vi "ORGINAL_drawLabel.vi"(0 "reference":refnum<class "StateTransitionEdge.lvclass">, 1 "graphics":refnum<class "Graphics.lvclass">, 5 "error in (no error)":errorcluster) -> (14 "reference out":refnum<class "StateTransitionEdge.lvclass">, 19 "error out":errorcluster)   [LabVIEW 2012, in "StateTransitionEdge.lvclass"]
doc: "private void drawLabel(Graphics2D g2)"
uses:
  <resource>/Framework/Providers/Open_GDS/UML/StateTransitionEdge_class/StateTransitionEdge.lvclass
  <resource>/Framework/Providers/Open_GDS/UML/Graphics_class/Graphics.lvclass
  <resource>/Framework/Providers/Open_GDS/UML/General/Point/Point Point2D.ctl
  <resource>/Framework/Providers/Open_GDS/UML/SegmentedLineEdge_class/SegmentedLineEdge.lvclass
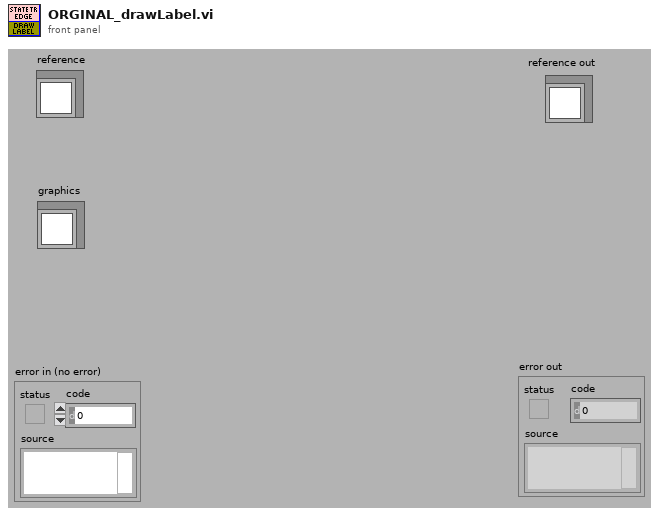
[diagram p1: front panel]
types:
  T1 = typedef "Point Point2D.ctl" = cluster{"x":dbl, "y":dbl}
  T2 = typedef "SegmentedLineEdge.lvclass/ObjectAttributes.ctl" = cluster{"lineStyle":refnum<class "LineStyle.lvclass">, "startArrowHead":refnum<class "ArrowHead.lvclass">, "endArrowHead":refnum<class "ArrowHead.lvclass">, "startLabel":string, "midLabel":string, "endLabel":string, "MidLabelOffset":T1, "SplitWire":bool}
  T3 = typedef "Rectangle Rectangle2D.ctl" = cluster{"x":dbl, "y":dbl, "width":dbl, "height":dbl}
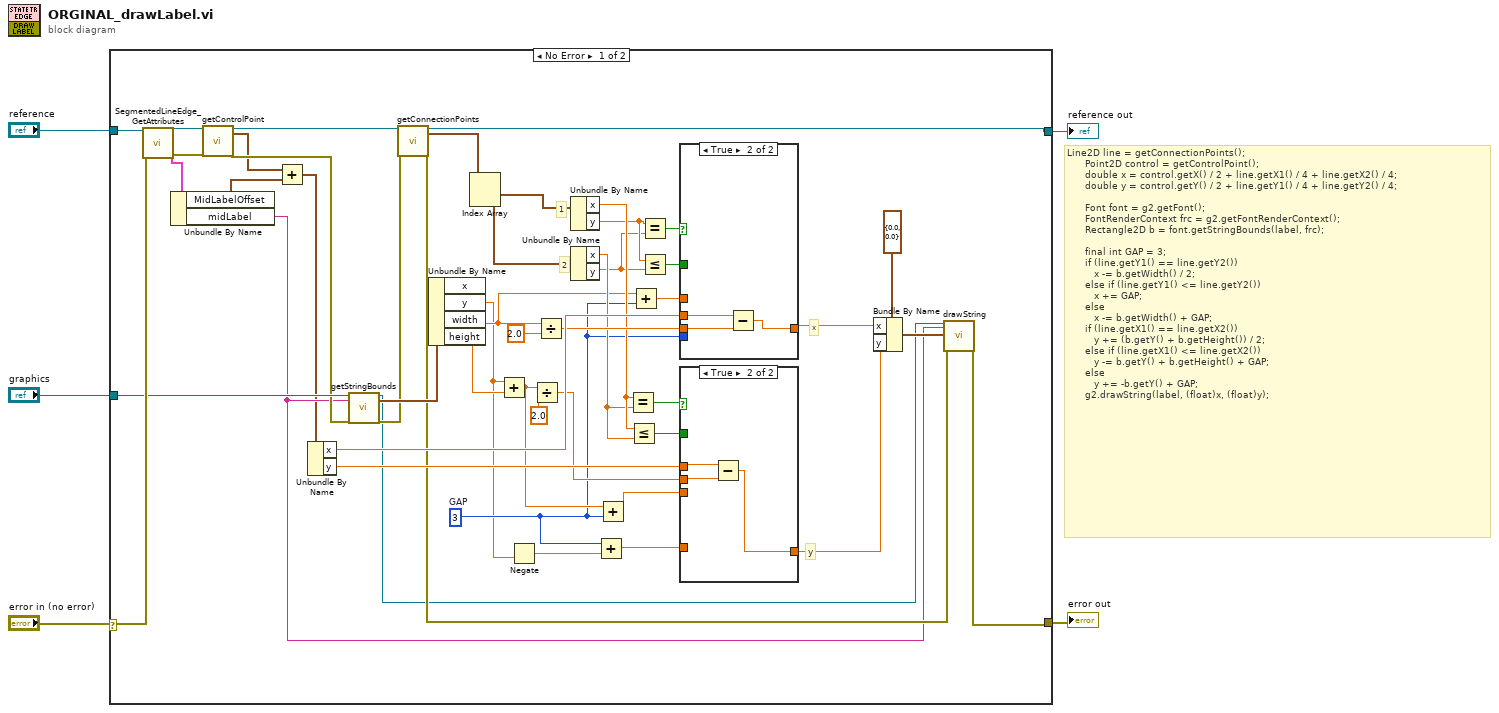
[diagram p0: block diagram]
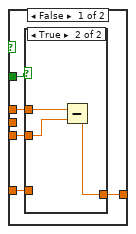
[diagram p2: hidden frame]
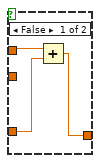
[diagram p3: hidden frame]
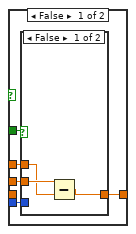
[diagram p4: hidden frame]
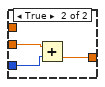
[diagram p5: hidden frame]
diagram:
  # "Line2D line = getConnectionPoints();\n      Point2D control = getControlPoint();\n      double x = control.getX() / 2 + line.getX1() / 4 + line.getX2() / 4;\n      double y = control.getY() / 2 + line.getY1() / 4 + line.getY2() / 4;\n\n      Font font = g2.getFont();\n      FontRenderContext frc = g2.getFontRenderContext();\n      Rectangle2D b = font.getStringBounds(label, frc);      \n\n      final int GAP = 3;\n      if (line.getY1() == line.getY2())\n         x -= b.getWidth() / 2;\n      else if (line.getY1() <= line.getY2())\n         x += GAP;\n      else\n         x -= b.getWidth() + GAP;\n      if (line.getX1() == line.getX2())\n         y += (b.getY() + b.getHeight()) / 2;\n      else if (line.getX1() <= line.getX2())\n         y -= b.getY() + b.getHeight() + GAP;\n      else\n         y += -b.getY() + GAP;\n      g2.drawString(label, (float)x, (float)y);"
  n1 = case shown="No Error" "error in (no error)" {
    selector: "error in (no error)" -> [w52 w82]
    tunnel: "reference" -> [w53 w83]
    tunnel: [w15 w82] -> w4
    tunnel: [w11 w83] -> w3
    tunnel: "graphics" -> [w49 _]
    frame No Error {
      w18 = 3  # GAP
      # "y"
      # "x"
      # "2"
      # "1"
      n2 = call <resource>:"SegmentedLineEdge_GetAttributes.vi"("reference in"=w53, "error in (no error)"=w52) -> ("reference out"=w51:refnum<class "StateTransitionEdge.lvclass">, "Data"=w6:T2, "error out"=w50:errorcluster)  [unwired: 14 in, 1 out]
      n3 = Unbundle By Name(w6) -> ("MidLabelOffset"=w7:T1, "midLabel"=w12:string)
      n4 = call <resource>:"getControlPoint.vi"("reference"=w51, "error in (no error)"=w50) -> ("reference out"=w36:refnum<class "StateTransitionEdge.lvclass">, "point"=w39:T1, "error out"=w48:errorcluster)  [unwired: 15 out]
      n5 = Add(x=w39, y=w7) -> (x+y=w8:T1)
      n6 = Unbundle By Name(w8) -> ("x"=w33:dbl, "y"=w31:dbl)
      n7 = call-dynamic "getStringBounds.vi"("reference"=w49, "text"=w12, "error in (no error)"=w48) -> ("reference out"=w13:refnum<class "Graphics.lvclass">, "bounds"=w47:T3, "error out"=w37:errorcluster)  [unwired: 14 in]
      n8 = call-dynamic "getConnectionPoints.vi"("reference"=w36, "error in (no error)"=w37) -> ("reference out"=w11:refnum<class "StateTransitionEdge.lvclass">, "line"=w38:T1[], "error out"=w14:errorcluster)  [unwired: 15 in]
      n9 = Unbundle By Name(w47) -> ("y"=w9:dbl, "width"=w17:dbl, "height"=w10:dbl)  [unwired: 1 out]
      n10 = Index Array(array=w38) -> (element #1=w35:T1, element #2=w34:T1)  [unwired: 2 in]
      n11 = Add(x=w9, y=w10) -> (x+y=w25:dbl)
      n12 = Negate(x=w9) -> (-x=w23:dbl)
      n13 = Divide(x=w25, y=2.0) -> (x/y=w29:dbl)
      n14 = Divide(x=w17, y=2.0) -> (x/y=w32:dbl)
      n15 = Unbundle By Name(w35) -> ("x"=w28:dbl, "y"=w21:dbl)
      n16 = Unbundle By Name(w34) -> ("x"=w27:dbl, "y"=w20:dbl)
      n17 = Add(x=w18, y=w23) -> (x+y=w22:dbl)
      n18 = Add(x=w25, y=w18) -> (x+y=w24:dbl)
      n19 = Equal?(x=w28, y=w27) -> (x = y?=w44:bool)
      n20 = Less Or Equal?(x=w28, y=w27) -> (x <= y?=w26:bool)
      n21 = Add(x=w17, y=w18) -> (x+y=w16:dbl)
      n22 = Equal?(x=w21, y=w20) -> (x = y?=w45:bool)
      n23 = Less Or Equal?(x=w21, y=w20) -> (x <= y?=w19:bool)
      n24 = case shown="True" w45 {
        tunnel: [w69 w79] -> w42
        tunnel: w33 -> [w71 w81]
        tunnel: w32 -> [_ w80]
        tunnel: w19 -> [w72 _]
        tunnel: w18 -> [w70 _]
        tunnel: w16 -> [w68 _]
        frame False {
          n25 = case shown="False" w72 {
            tunnel: w71 -> [w75 w78]
            tunnel: w70 -> [_ w77]
            tunnel: [w73 w76] -> w69
            tunnel: w68 -> [w74 _]
            frame False {
              n26 = Subtract(x=w75, y=w74) -> (x-y=w73:dbl)
            }
            frame True {
              n27 = Add(x=w78, y=w77) -> (x+y=w76:dbl)
            }
          }
        }
        frame True {
          n28 = Subtract(x=w81, y=w80) -> (x-y=w79:dbl)
        }
      }
      n29 = case shown="True" w44 {
        tunnel: [w56 w65] -> w41
        tunnel: w31 -> [w57 w67]
        tunnel: w29 -> [_ w66]
        tunnel: w26 -> [w58 _]
        tunnel: w24 -> [w55 _]
        tunnel: w22 -> [w54 _]
        frame False {
          n30 = case shown="True" w58 {
            tunnel: w57 -> [w61 w64]
            tunnel: [w60 w63] -> w56
            tunnel: w55 -> [_ w62]
            tunnel: w54 -> [w59 _]
            frame False {
              n31 = Add(x=w61, y=w59) -> (x+y=w60:dbl)
            }
            frame True {
              n32 = Subtract(x=w64, y=w62) -> (x-y=w63:dbl)
            }
          }
        }
        frame True {
          n33 = Subtract(x=w67, y=w66) -> (x-y=w65:dbl)
        }
      }
      n34 = Bundle By Name(cluster=T1 {"x"=0.0, "y"=0.0} ("textPos"), "x"=w42, "y"=w41) -> (w40:T1)
      n35 = call-dynamic "drawString.vi"("reference"=w13, "text"=w12, "textPos"=w40, "error in (no error)"=w14) -> ("error out"=w15:errorcluster)  [unwired: 14 in, 1 out]
    }
    frame Error {
    }
  }
  "reference out" <- w3
  "error out" <- w4
